vi "1. Work with ultrasensor and servo motor.vi"() -> ()   [LabVIEW 2020]
uses:
  <vilib>/robotics/Starter Kit/2.0/9632 Host Interface/NI_Robotics_Starter Kit Host_9632_2.0.lvclass
panel:
  in  "stop":bool
  out "Waveform Chart":dbl(graph)
  in  "Servo angle (deg)":dbl(slide) scale=-65.0..65.0
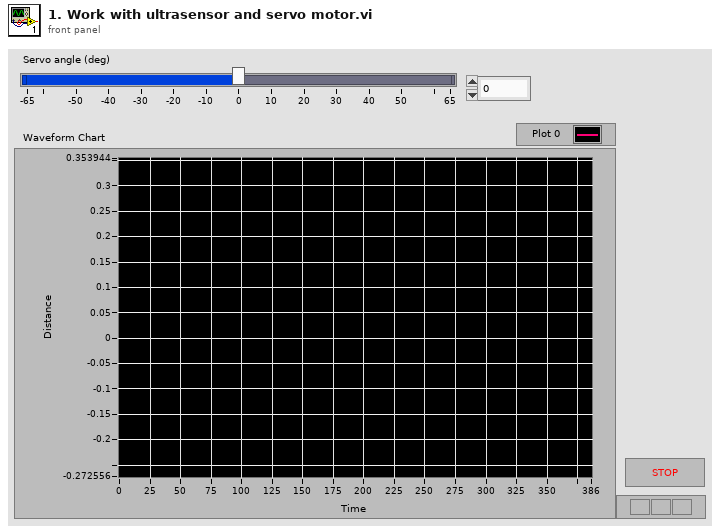
[diagram p1: front panel]
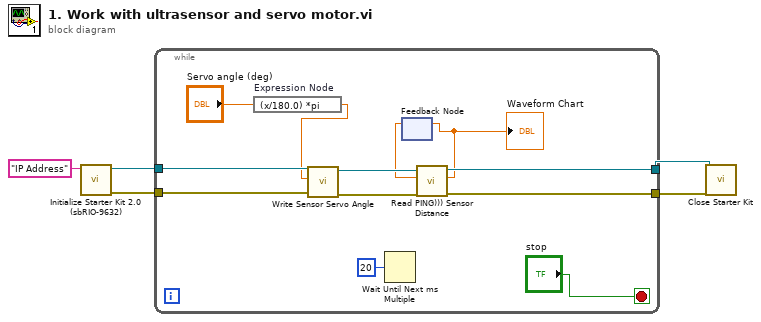
[diagram p0: block diagram]
diagram:
  n1 = call <vilib>:"Initialize Starter Kit 2.0 (sbRIO-9632).vi"("IP address (\"\")"="IP Address" ("IP address (\"\")")) -> ("error out"=w3:errorcluster, "FPGA starter kit host 2.0 out"=w4:refnum<class "NI_Robotics_Starter Kit Host_9632_2.0.lvclass">)  [unwired: 9 in]
  n2 = while {
    tunnel: w4 -> [w16]
    tunnel: w3 -> [w15]
    tunnel: [w10] -> w2
    tunnel: [w9] -> w1
    stop <- "stop" stop-if-true
    n3 = expression code="(x/180.0) *pi"("Servo angle (deg)") -> (w14:dbl)
    n4 = call <vilib>:"Write Sensor Servo Angle.vi"("error in (no error)"=w15, "ccw servo angle (rad)"=w14, "starter kit host in"=w16) -> ("error out"=w12:errorcluster, "starter kit host out"=w13:refnum<class "NI_Robotics_Starter Kit Host_9632_2.0.lvclass">)  [unwired: 7 in]
    n5 = Wait Until Next ms Multiple(millisecond multiple=u32 20) -> ()  [unwired: 1 out]
    n6 = feedback #1() -> (w6:dbl)  [unwired: 1 in]
    n7 = call <vilib>:"Read PING))) Sensor Distance.vi"("error in (no error)"=w12, "default distance (NaN)"=w6, "starter kit host in"=w13) -> ("error out"=w9:errorcluster, "distance (m)"=w7:dbl, "starter kit host out"=w10:refnum<class "NI_Robotics_Starter Kit Host_9632_2.0.lvclass">)  [unwired: 5 in, 1 out]
    "Waveform Chart" <- w7
    n8 = feedback-in #1(w7) -> ()
  }
  n9 = call-dynamic "Close Starter Kit.vi"("error in (no error)"=w1, "starter kit host in"=w2) -> ()  [unwired: 9 in, 1 out]
